vi "GUI_laptop v2.vi"() -> ()   [LabVIEW 2019]
uses:
  <vilib>/Platform/TimedLoop/XDataNode/wakeup.ctl
  <vilib>/Platform/TimedLoop/XDataNode/XDNodeRunTimeDep.lvlib
  <vilib>/Platform/TimedLoop/XDataNode/nitl_modes.ctl
  <vilib>/Platform/TimedLoop/XDataNode/timing_clust.ctl
  <vilib>/platform/TimedLoop/XDataNode/XDataNode.xnode
  <vilib>/Native 3D Graph/xcontrol/3DPC_SurfacePlot.xctl
  <vilib>/Analysis/NI_AALBLAS.lvlib
  <vilib>/Instr/_visa.llb/VISA Configure Serial Port (Instr).vi
  <vilib>/Analysis/BLAS.llb/dnrm2 - Vector 2-Norm (DBL).vi
  <vilib>/Utility/file.llb/Write Delimited Spreadsheet (DBL).vi
panel:
  in  "L5 bound":dbl
  in  "L4 bound":dbl
  in  "L3 bound":dbl
  in  "L2 bound":dbl
  in  "L1 bound":dbl
  in  "Epsilon radius":dbl
  out "3D Graph":refnum<class "Base Datatype.lvclass">[](xcontrol)
  in  "Num of Points":i32
  in  "z bound":dbl
  in  "y bound":dbl
  in  "x bound":dbl
  in  "Stop":bool
  in  "Round Decimals":dbl format="%#_15g"
  in  "Save  Data":bool
  in  "Save Path":path
  out "error out":errorcluster
  in  "baud rate":u32=9600
  in  "VISA resource name":refnum<visa-resource-name>
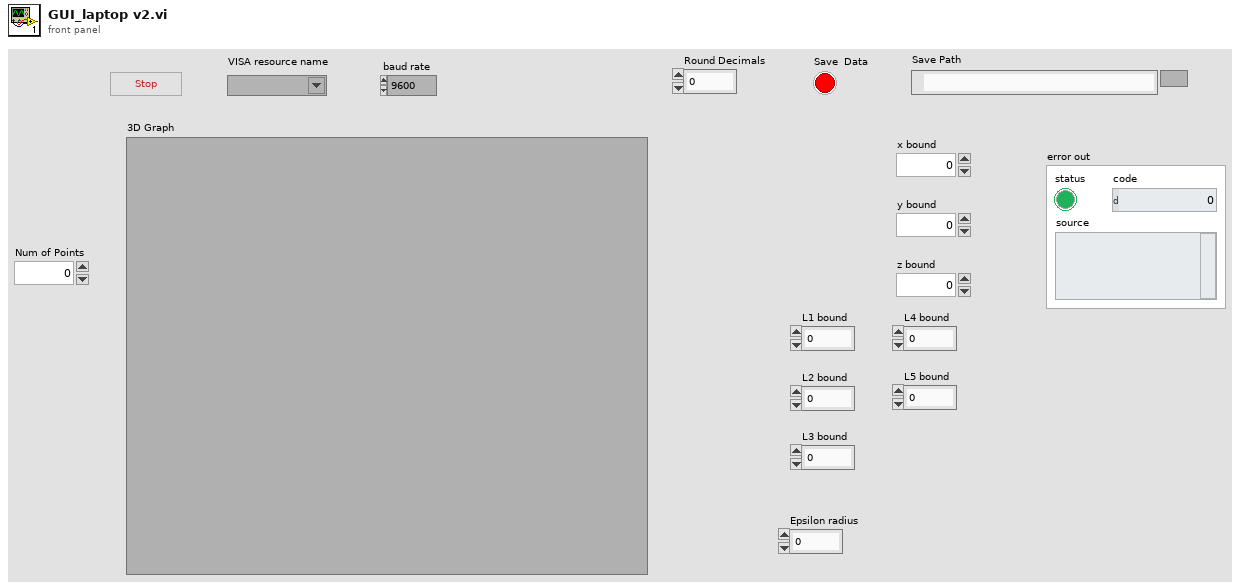
[diagram p1: front panel]
types:
  T1 = typedef "XDNodeRunTimeDep.lvlib/timing_clust.ctl" = cluster{"Expected End [f-1]":u64, "Actual End [f-1]":u64, "Finished Late? [f-1]":bool, "Expected End [i-1]":u64, "Actual End [i-1]":u64, "Finished Late? [i-1]":bool, "Expected Start [i]":u64, "Actual Start [i]":u64, "Expected Start [f]":u64, "Actual Start [f]":u64, "Source Name":string, "Structure Name":string, "Period":i64, "Deadline":i64, "Offset":i64, "Start":i64, "Priority":i32, "Timeout":i32, "Mode":T2, "Wakeup Reason":T3, "Error":errorcluster, "Source Type":string, "Secondary Source Type":string, "Global End Time":u64, "Global Start Time":u64, "Frame Duration":u64, "Iteration Duration":u64, "Assigned CPU":i32, "I/O Scan Engine Mode":u32}
  T2 = typedef "XDNodeRunTimeDep.lvlib/nitl_modes.ctl" = enum32{"No Change", "Process missed periods, maintain original phase", "Discard missed periods, maintain original phase", "Process missed periods, ignore original phase", "Discard missed periods, ignore original phase"}
  T3 = typedef "XDNodeRunTimeDep.lvlib/wakeup.ctl" = enum32{"Normal", "Aborted", "Asynchronous wakeup", "Timing source error", "Timed loop error", "Timeout"}
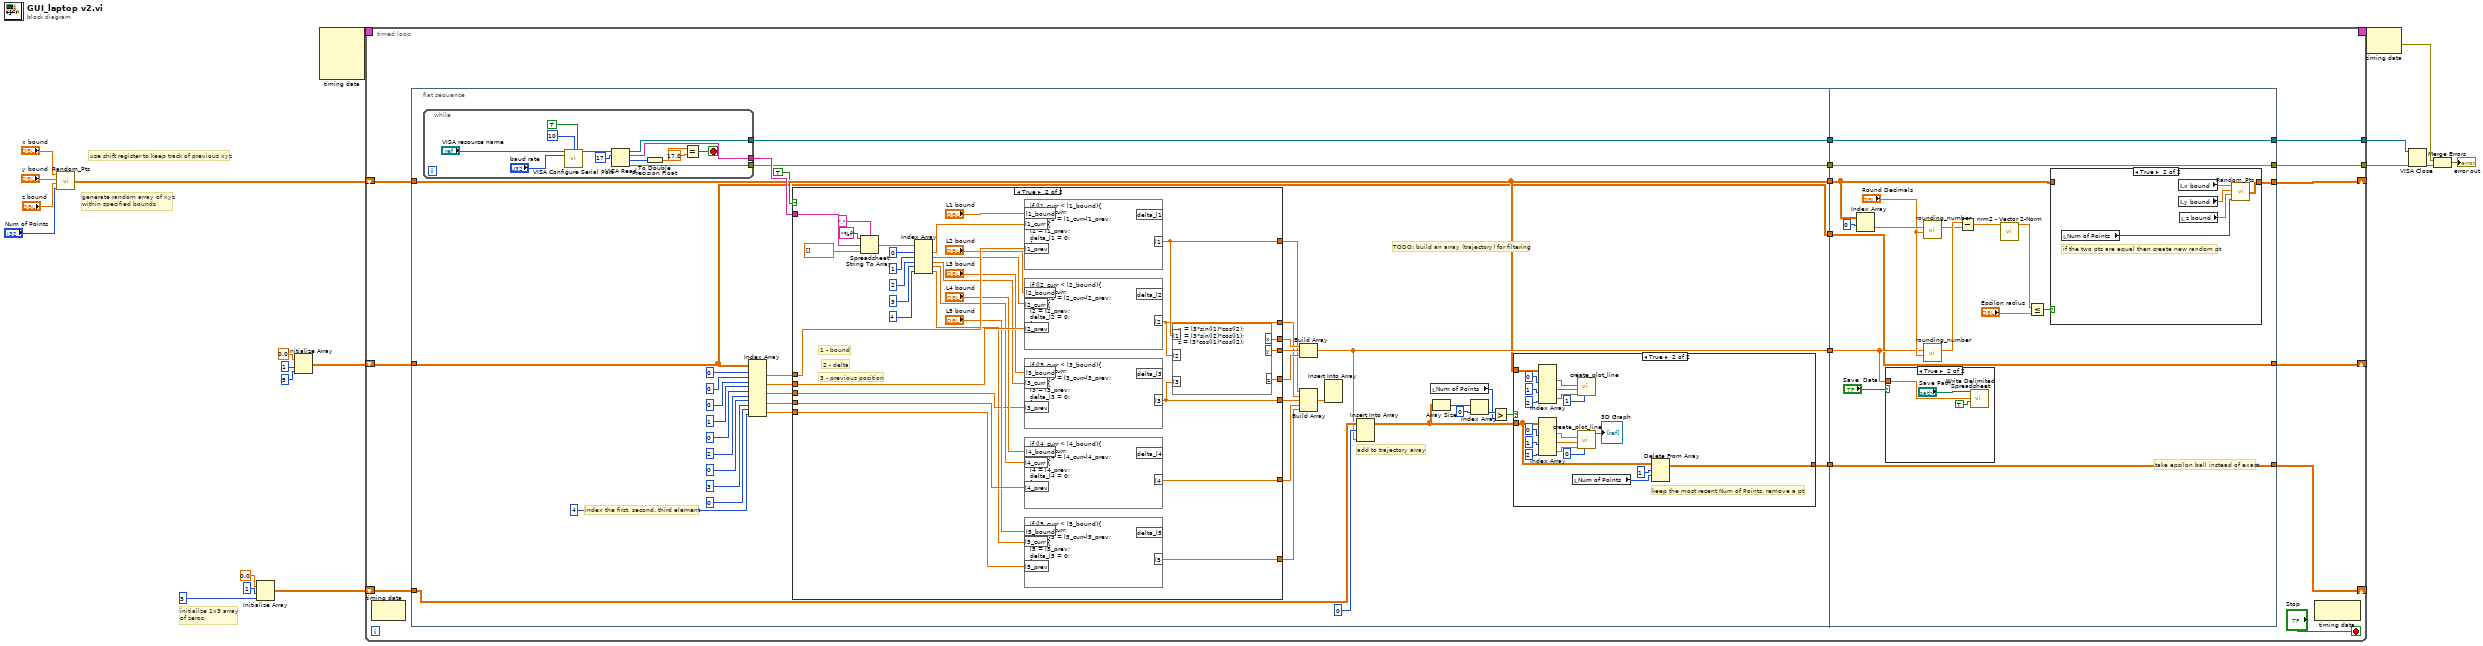
[diagram p0: block diagram]
diagram:
  # "use shift register to keep track of previous xyz"
  # "generate random array of xyz\nwithin specified bounds"
  # "initialize 1x3 array \nof zeros"
  n1 = call "Random_Pts.vi"("Num of Points"="Num of Points", "z bound"="z bound", "y bound"="y bound", "x bound"="x bound") -> ("appended array"=w6:dbl[][])
  n2 = Initialize Array(0.0 ("element"), 1 ("dimension size"), 3 ("dimension size")) -> (w13:dbl[][])
  n3 = Initialize Array(0.0 ("element"), 1 ("dimension size"), 5 ("dimension size")) -> (w1:dbl[][])
  n4 = node-c288() -> (w20:T1)  [unwired: 4 in]
  n5 = timed-loop {
    tunnel: [w34] -> w15
    tunnel: [w33] -> w14
    shift-right: [w32] -> _
    shift-left: w13 -> [w31]
    timing: w20 -> [_]
    timing-out: [_] -> w19
    shift-right: [w24] -> _
    shift-left: w6 -> [w26]
    shift-right: [w21] -> _
    shift-left: w1 -> [w23]
    stop <- "Stop" stop-if-true
    n6 = node-c288() -> ()  [unwired: 1 in, 1 out]
    n7 = flat-sequence {
      tunnel: w31 -> [w59]
      tunnel: [w52] -> w30
      tunnel: [w76] -> w29
      tunnel: [w53] -> w28
      tunnel: [w58] -> w27
      tunnel: w26 -> [w55]
      tunnel: [w55] -> w25
      tunnel: w23 -> [w38]
      tunnel: [w38] -> w22
      tunnel: w30 -> [w166]
      tunnel: w29 -> [w165]
      tunnel: w28 -> [w164]
      tunnel: w27 -> [w158]
      tunnel: w25 -> [w160]
      tunnel: [w166] -> w34
      tunnel: [w165] -> w33
      tunnel: [w164] -> w32
      tunnel: [w159] -> w24
      tunnel: [w150] -> w21
      tunnel: w22 -> [w150]
      frame #0 {
        # "TODO: build an array (trajectory) for filtering"
        # "add to trajectory array"
        # "index the first, second, third element"
        n8 = while {
          tunnel: [w148] -> w77
          tunnel: [w143] -> w76
          tunnel: [w137] -> w52
          stop <- w147 stop-if-true
          n9 = call-poly "VISA Configure Serial Port"("VISA resource name"="VISA resource name", "termination char\n(0xA = '\\n' = LF)"=u8 10 ("termination char\n(0xA = '\\n' = LF)"), "Enable Termination\nChar (T)"=TRUE ("Enable Termination\nChar (T)"), "baud rate (9600)"="baud rate") -> ("VISA resource name out"=w138:refnum<visa-resource-name>)  [unwired: 10 in, 1 out]
          n10 = VISA Read(VISA resource name=w138, byte count=u32 17) -> (VISA resource name out=w137:refnum<visa-resource-name>, read buffer=w148:string, return count=w145:u32, error out=w143:errorcluster)  [unwired: 1 in]
          n11 = To Double Precision Float(number=w145) -> (double precision float=w144:dbl)
          n12 = Equal?(x=w144, y=17.0 ("char count")) -> (x = y?=w147:bool)
        }
        n13 = Index Array(array=w38, index (row) #1=0 ("disabled index (row)"), index (col) #1=0 ("disabled index (col)"), index (row) #2=0 ("disabled index (row)"), index (col) #2=1 ("disabled index (col)"), index (row) #3=0 ("disabled index (row)"), index (col) #3=2 ("disabled index (col)"), index (row) #4=0 ("disabled index (row)"), index (col) #4=3 ("disabled index (col)"), index (row) #5=0 ("disabled index (row)"), index (col) #5=4 ("disabled index (col)")) -> (element #1=w69:dbl, element #2=w67:dbl, element #3=w68:dbl, element #4=w47:dbl, element #5=w46:dbl)
        n14 = case shown="True" TRUE {
          tunnel: w77 -> [_ w115]
          tunnel: w69 -> [w82 w111]
          tunnel: w68 -> [w80 w94]
          tunnel: w67 -> [w81 w104]
          tunnel: [_ w90] -> w63
          tunnel: [_ w88] -> w62
          tunnel: [_ w89] -> w61
          tunnel: w47 -> [w79 w99]
          tunnel: w46 -> [w78 w98]
          tunnel: [w82 w87] -> w44
          tunnel: [w81 w86] -> w43
          tunnel: [w80 w85] -> w42
          tunnel: [w79 w84] -> w41
          tunnel: [w78 w83] -> w40
          frame False {
            # "TODO: work on combining this and Zhantao's xyz reading"
          }
          frame True {
            # "2 - delta"
            # "1 - bound"
            # "3 - previous position"
            n15 = Spreadsheet String To Array(delimiter (Tab)=",", format string="%f", spreadsheet string=w115, array type (2D Dbl)=dbl[] []) -> (array=w107:dbl[])
            n16 = Index Array(array=w107, index #1=0 ("index"), index #2=1 ("index"), index #3=2 ("index"), index #4=3, index #5=4) -> (element #1=w96:dbl, element #2=w95:dbl, element #3=w93:dbl, element #4=w92:dbl, element #5=w91:dbl)
            n17 = formula code="if (l1_curr < l1_bound){\nl1 = l1_curr;\ndelta_l1 = l1_curr-l1_prev;\n}else{\nl1 = l1_prev;\ndelta_l1 = 0;\n}"("l1_bound"="L1 bound", "l1_prev"=w111, "l1_curr"=w96) -> ("l1"=w87:dbl)  [unwired: 1 out]
            n18 = formula code="if (l2_curr < l2_bound){\nl2 = l2_curr;\ndelta_l2 = l2_curr-l2_prev;\n}else{\nl2 = l2_prev;\ndelta_l2 = 0;\n}"("l2_bound"="L2 bound", "l2_prev"=w104, "l2_curr"=w95) -> ("l2"=w86:dbl)  [unwired: 1 out]
            n19 = formula code="if (l3_curr < l3_bound){\nl3 = l3_curr;\ndelta_l3 = l3_curr-l3_prev;\n}else{\nl3 = l3_prev;\ndelta_l3 = 0;\n}"("l3_bound"="L3 bound", "l3_prev"=w94, "l3_curr"=w93) -> ("l3"=w85:dbl)  [unwired: 1 out]
            n20 = formula code="if (l4_curr < l4_bound){\nl4 = l4_curr;\ndelta_l4 = l4_curr-l4_prev;\n}else{\nl4 = l4_prev;\ndelta_l4 = 0;\n}"("l4_bound"="L4 bound", "l4_prev"=w99, "l4_curr"=w92) -> ("l4"=w84:dbl)  [unwired: 1 out]
            n21 = formula code="if (l5_curr < l5_bound){\nl5 = l5_curr;\ndelta_l5 = l5_curr-l5_prev;\n}else{\nl5 = l5_prev;\ndelta_l5 = 0;\n}"("l5_bound"="L5 bound", "l5_prev"=w98, "l5_curr"=w91) -> ("l5"=w83:dbl)  [unwired: 1 out]
            n22 = formula code="x = l3*sin(l1)*cos(l2);\ny = l3*sin(l2)*cos(l1);\nz = l3*cos(l1)*cos(l2);"("l1"=w87, "l2"=w86, "l3"=w85) -> ("x"=w90:dbl, "y"=w89:dbl, "z"=w88:dbl)
          }
        }
        n23 = Build Array(w63, w61, w62) -> (w58:dbl[])
        n24 = Build Array(w44, w43, w42, w41, w40) -> (w39:dbl[])
        n25 = Insert Into Array(new element=w39) -> ()  [unwired: 3 in, 1 out]
        n26 = Insert Into Array(array=w59, index (row)=0, new element=w58) -> (w56:dbl[][])  [unwired: 1 in]
        n27 = local read "Num of Points"() -> (w57:i32)
        n28 = Array Size(array=w56) -> (size(s)=w60:i32[])
        n29 = Index Array(array=w60, index=0) -> (element=w64:i32)
        n30 = Greater?(x=w64, y=w57) -> (0:w54:bool)
        n31 = case shown="True" w54 {
          tunnel: w56 -> [w116 w132]
          tunnel: [w116 w131] -> w53
          tunnel: w55 -> [_ w130]
          frame False {
          }
          frame True {
            # "keep the most recent Num of Points, remove a pt"
            n32 = Index Array(array=w130, index (col) #1=0 ("disabled index (col)"), index (col) #2=1 ("index (col)"), index (col) #3=2 ("index (col)")) -> (element #1=w120:dbl[], element #2=w119:dbl[], element #3=w118:dbl[])  [unwired: 3 in]
            n33 = Index Array(array=w132, index (col) #1=0 ("disabled index (col)"), index (col) #2=1 ("index (col)"), index (col) #3=2 ("index (col)")) -> (element #1=w123:dbl[], element #2=w122:dbl[], element #3=w121:dbl[])  [unwired: 3 in]
            n34 = local read "Num of Points"() -> (w126:i32)
            n35 = call <vilib>:"create_plot_line.vi"("plot ID"=1, "z vector"=w118, "y vector"=w119, "x vector"=w120) -> ()  [unwired: 1 in, 7 out]
            n36 = call <vilib>:"create_plot_line.vi"("plot ID"=0, "z vector"=w121, "y vector"=w122, "x vector"=w123) -> ("plots out"=→"3D Graph":refnum<class "Base Datatype.lvclass">[])  [unwired: 1 in, 6 out]
            n37 = Delete From Array(array=w132, length=1, index (row)=w126) -> (array with subset deleted=w131:dbl[][])  [unwired: 1 in, 1 out]
          }
        }
      }
      frame #1 {
        # "take epsilon ball instead of exact"
        n38 = Index Array(array=w160, index (row)=0) -> (element=w162:dbl[])  [unwired: 1 in]
        n39 = case shown="True" "Save  Data" {
          tunnel: w158 -> [_ w167]
          frame False {
          }
          frame True {
            n40 = call-poly <vilib>:"Write Delimited Spreadsheet.vi"("file path (dialog if empty)"="Save Path", "1D data"=w167, "append to file? (new file:F)"=TRUE) -> ()  [unwired: 11 in, 2 out]
          }
        }
        n41 = call "rounding_number.vi"("power of ten"="Round Decimals", "Array"=w162) -> ("rounded"=w153:dbl[])  [unwired: 9 in]
        n42 = call "rounding_number.vi"("power of ten"="Round Decimals", "Array"=w158) -> ("rounded"=w154:dbl[])  [unwired: 9 in]
        n43 = Subtract(x=w154, y=w153) -> (x-y=w152:dbl[])
        n44 = call-poly <vilib>:"nrm2 - Vector 2-Norm.vi"("x"=w152) -> ("dnrm2"=w151:dbl)  [unwired: 9 in, 1 out]
        n45 = Less Or Equal?(x=w151, y="Epsilon radius") -> (x <= y?=w155:bool)
        n46 = case shown="True" w155 {
          tunnel: w160 -> [w170 _]
          tunnel: [w170 w171] -> w159
          frame False {
          }
          frame True {
            # "if the two pts are equal then create new random pt"
            n47 = local read "Num of Points"() -> (w172:i32)
            n48 = local read "x bound"() -> (w175:dbl)
            n49 = local read "y bound"() -> (w174:dbl)
            n50 = local read "z bound"() -> (w173:dbl)
            n51 = call "Random_Pts.vi"("Num of Points"=w172, "z bound"=w173, "y bound"=w174, "x bound"=w175) -> ("appended array"=w171:dbl[][])
          }
        }
      }
    }
    n52 = node-c288() -> ()  [unwired: 1 in, 1 out]
  }
  n53 = node-c288(w19) -> (w12:errorcluster)
  n54 = VISA Close(VISA resource name=w15, error in (no error)=w14) -> (error out=w11:errorcluster)
  n55 = Merge Errors(w12, w11) -> (→"error out":errorcluster)
